vi "qPUN.vi"(0 "System no.":i32=1 min=1 max=4 step=1, 2 "Axes to query":string[](array[string]), 3 "All Axes?":bool, 4 "Axis Identifier?":bool=TRUE, 5 "error in":errorcluster) -> (14 "Position unit":string[](array[string]), 19 "error out":errorcluster)   [LabVIEW 2026]
doc: "Returns the name of the connected stage for queried axes.\n\nC-413, E-712, E-725,E-727,E-753: If All axes? = TRUE, then Axis identifier? can be FALSE. \n\nC-886, E-754: If All axes? = TRUE, then Axis identifier? can be FALSE. \n\nC-887, F-206, M-8X0: If All axes? = TRUE, then Axis identifier? can be FALSE. Only for GCS syntax version = GCS 2.0 or higher (check with CSV?.vi. If CSV?.vi is not supported, syntax version is GCS 1.0)."
panel:
  # "Returns the name of the current position unit for queried axes."
  # "If all axes: use"
  # "Query"
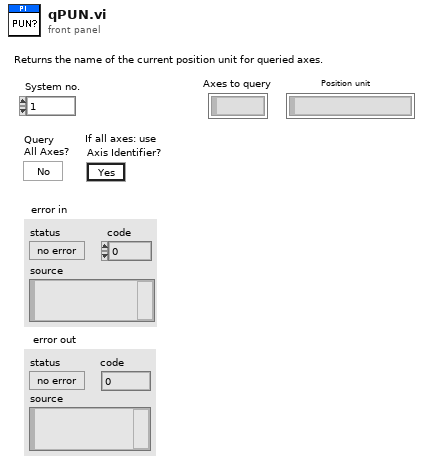
[diagram p1: front panel]
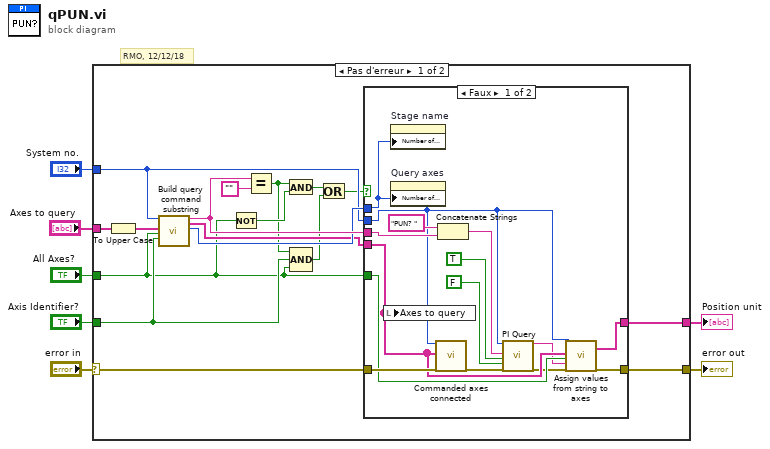
[diagram p0: block diagram]
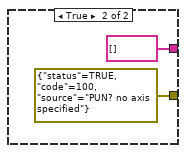
[diagram p2: hidden frame]
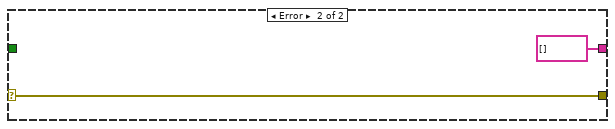
[diagram p3: hidden frame]
diagram:
  # "RMO, 12/12/18"
  n1 = case shown="Pas d'erreur" "error in" {
    selector: "error in" -> [w8 w42]
    tunnel: "Axes to query" -> [w24 _]
    tunnel: [w10 w42] -> w6
    tunnel: "System no." -> [w19 _]
    tunnel: "Axis Identifier?" -> [w14 _]
    tunnel: "All Axes?" -> [w13 _]
    tunnel: [w11 string[] [] ("Strings")] -> w2
    frame No Error {
      n2 = To Upper Case(1:w24) -> (0:w22:string[])
      n3 = call "Build query command substring.vi"("System no."=w19, "Axes to query in"=w22, "Query\nAll axes?"=w13, "For all axes: use\nAxis identifier?"=w14) -> ("Command substring"=w21:string, "Axes to query out"=w18:string[], "Number of rows"=w20:u32)  [unwired: 2 in, 11 out]
      n4 = Not(x=w13) -> (.not. x?=w17:bool)
      n5 = Equal?(x=w21, y="" ("x")) -> (x = y?=w15:bool)
      n6 = And(x=w15, y=w17) -> (x .and. y?=w16:bool)
      n7 = Compound Arithmetic op=AND(w15, w14, w13) -> (w12:bool)
      n8 = Or(x=w16, y=w12) -> (x .or. y?=w9:bool)
      n9 = case shown="Faux" w9 {
        tunnel: w8 -> [w36 _]
        tunnel: w21 -> [w35 _]
        tunnel: w20 -> [w34 _]
        tunnel: w19 -> [w33 _]
        tunnel: w18 -> [w32 _]
        tunnel: w13 -> [w31 _]
        tunnel: [w30 string[] [] ("Strings")] -> w11
        tunnel: [w28 errorcluster {"status"=TRUE, "code"=100, "source"="PUN? no axis specified"} ("error out")] -> w10
        frame False {
          n10 = local write "Axes to query"(w32) -> ()
          n11 = property on="Stage name" class="Tabl (strict)"("Number of Rows"=w34) -> ()  [unwired: 2 in, 2 out]
          n12 = property on="Query axes" class="Tabl (strict)"("Number of Rows"=w34) -> ()  [unwired: 2 in, 2 out]
          n13 = call "Commanded axes connected.vi"("System no."=w33, "Commanded axes"=w32, "error in"=w36) -> ("error out"=w29:errorcluster)  [unwired: 1 in, 15 out]
          n14 = Concatenate Strings("PUN? ", w35) -> (w37:string)
          n15 = call "PI Query.vi"("System no."=w33, "String to send"=w37, "Attach termination char.?"=TRUE ("Attach Linefeed?"), "Strip spaces?"=FALSE, "error in"=w29) -> ("String read"=w26:string, "error out"=w25:errorcluster)  [unwired: 2 in, 11 out]
          n16 = call "Assign values from string to axes.vi"("System no."=w33, "Queried axes"=w32, "All axes queried?"=w31, "Input String"=w26, "error in"=w25) -> ("Strings"=w30:string[], "error out"=w28:errorcluster)  [unwired: 4 in, 9 out]
        }
        frame True {
        }
      }
    }
    frame Error {
    }
  }
  "error out" <- w6
  "Position unit" <- w2
